vi "KeeperRole.vi"(7 "First call?":bool=TRUE, 8 "error in (no error)":errorcluster, 9 "Robot in":refnum<class "Robot.lvclass">, 10 "Game in":refnum<class "Game.lvclass">, 11 "KeeperRole in":refnum<class "KeeperRole.lvclass">) -> (0 "error out":errorcluster, 2 "Robot out":refnum<class "Robot.lvclass">, 3 "KeeperRole out":refnum<class "KeeperRole.lvclass">)   [LabVIEW 2024, in "KeeperRole.lvclass"]
uses:
  KeeperRole.lvclass
  C:/Users/ROBOIME2/Documents/SSL ROBOIME/SSL_AI/Role_class/Role.lvclass
  Robot_class/Robot.lvclass
  Game_class/Game.lvclass
  Role_class/Role.lvclass/Role.ctl
  DefendGoalTactic_class/Read States.vi
  Role_class/Read Tacticbook.vi
  Role_class/Read tactic_index.vi
  Role_class/Write Tacticbook.vi
  Role_class/Write tactic_index.vi
  Tacticbook_class/Tacticbook.lvclass
  DefendGoalTactic_class/DefendGoalTactic.lvclass
panel:
  out "Game out":refnum<class "Game.lvclass">
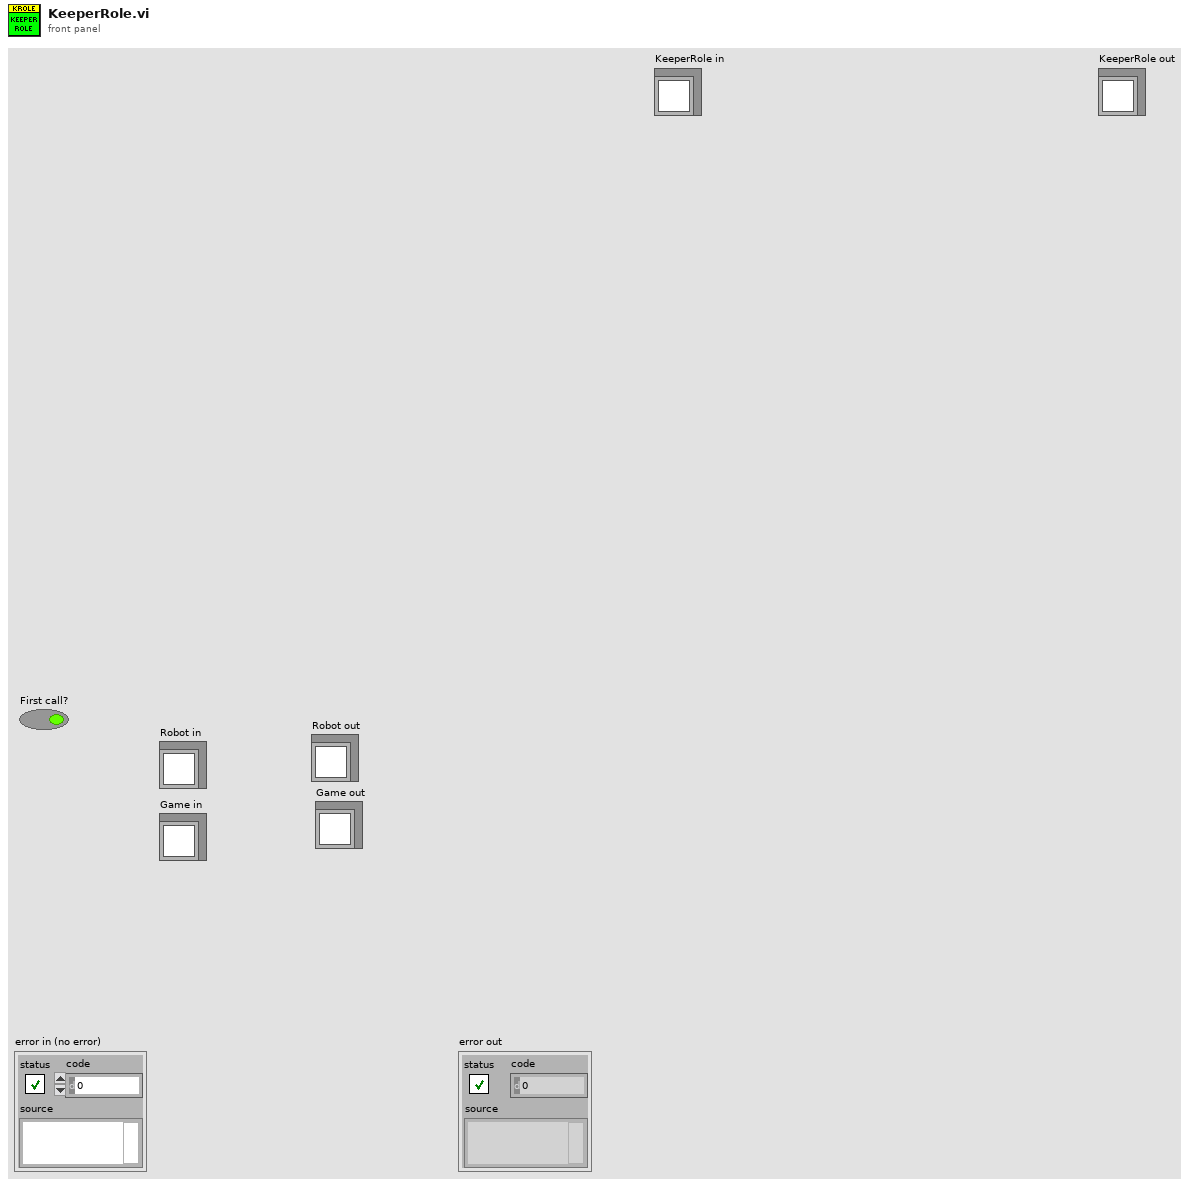
[diagram p1: front panel]
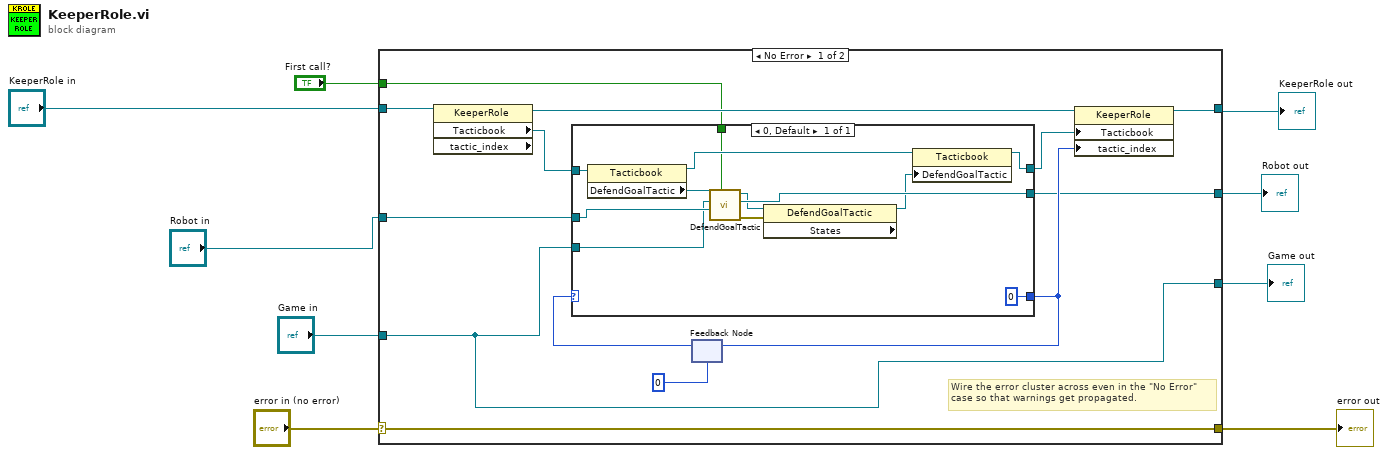
[diagram p0: block diagram]
diagram:
  n1 = case shown="No Error" "error in (no error)" {
    selector: "error in (no error)" -> [w22 w38]
    tunnel: [w22 w38] -> w8
    tunnel: [w20 w37] -> w2
    tunnel: "KeeperRole in" -> [w21 w37]
    tunnel: "Robot in" -> [w14 w36]
    tunnel: [w13 w36] -> w7
    tunnel: [w11 w35] -> w6
    tunnel: "Game in" -> [w11 w35]
    tunnel: "First call?" -> [w10 _]
    frame No Error {
      # "Wire the error cluster across even in the \"No Error\"\ncase so that warnings get propagated."
      n2 = property class="KeeperRole" props=["Tacticbook", "tactic_index"](reference=w21) -> (reference out=w19:refnum<class "KeeperRole.lvclass">, "Tacticbook"=w16:refnum<class "Tacticbook.lvclass">)  [unwired: 1 in, 2 out]
      n3 = feedback #1(0) -> (w17:i32)
      n4 = case shown="0, Default" w17 {
        tunnel: [0] -> w15
        tunnel: w16 -> [w34]
        tunnel: w14 -> [w27]
        tunnel: [w33] -> w13
        tunnel: [w29] -> w12
        tunnel: w11 -> [w25]
        tunnel: w10 -> [w23]
        frame 0, Default {
          n5 = property class="Tacticbook"(reference=w34) -> (reference out=w31:refnum<class "Tacticbook.lvclass">, "DefendGoalTactic"=w28:refnum<class "DefendGoalTactic.lvclass">)  [unwired: 1 in, 1 out]
          n6 = call "DefendGoalTactic.vi"("First call?"=w23, "Robot"=w27, "Game"=w25, "DefendGoalTactic in"=w28) -> ("error out"=w32:errorcluster, "Robot out"=w33:refnum<class "Robot.lvclass">, "DefendGoalTactic out"=w26:refnum<class "DefendGoalTactic.lvclass">)  [unwired: 5 in]
          n7 = property class="DefendGoalTactic" props=["States"](reference=w26, error in=w32) -> (reference out=w30:refnum<class "DefendGoalTactic.lvclass">)  [unwired: 2 out]
          n8 = property class="Tacticbook"(reference=w31, "DefendGoalTactic"=w30) -> (reference out=w29:refnum<class "Tacticbook.lvclass">)  [unwired: 1 in, 1 out]
        }
      }
      n9 = feedback-in #1(w15) -> ()
      n10 = property class="KeeperRole"(reference=w19, "Tacticbook"=w12, "tactic_index"=w15) -> (reference out=w20:refnum<class "KeeperRole.lvclass">)  [unwired: 1 in, 1 out]
    }
    frame Error {
    }
  }
  "KeeperRole out" <- w2
  "error out" <- w8
  "Robot out" <- w7
  "Game out" <- w6
